vi "generate default line.vi"(8 "error in":errorcluster, 11 "operations table":T2) -> (0 "error out":errorcluster, 2 "line":T1)   [LabVIEW 2013, in "Modbus Slave editor node.lvclass"]
doc: "Platypus Framework 1.0.1.65\nNI Systems Engineering - National Instruments"
uses:
  Modbus Slave editor node.lvclass
  table reference.ctl
  table line.ctl
  <vilib>/NI/TBM Modules/modbus slave/module channel/Modbus Module Channel.lvclass
  <vilib>/NI/Tag Bus/tag/Data Type.ctl
  <vilib>/NI/TBM Modules/modbus slave/module channel/data bank type.ctl
  <vilib>/NI/Tag Bus/tag/tag descriptor.lvclass/tag descriptor.ctl
  <vilib>/NI/TBM Modules/modbus slave/module channel/Modbus Module Channel.lvclass/Modbus Module Channel.ctl
  <vilib>/NI/Tag Bus/tag/write tag name.vi
  <vilib>/NI/Tag Bus/tag/write data type.vi
  <vilib>/NI/TBM Modules/modbus slave/module channel/Write modbus type.vi
  <vilib>/NI/TBM Modules/modbus slave/module channel/Write starting address.vi
  <vilib>/NI/Tag Bus/tag/tag descriptor.lvclass
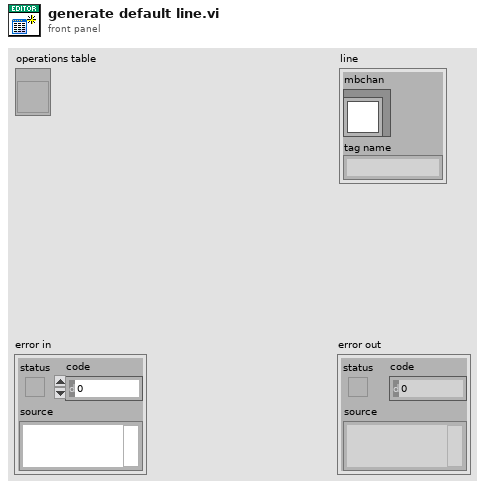
[diagram p1: front panel]
types:
  T1 = typedef "Modbus Slave editor node.lvclass/table line.ctl" = cluster{"mbchan":refnum<class "Modbus Module Channel.lvclass">, "tag name":string}
  T2 = typedef "Modbus Slave editor node.lvclass/table reference.ctl" = refnum<vi>
  T3 = typedef "Modbus Module Channel.lvclass/data bank type.ctl" = enum16{"coils", "discrete inputs", "input registers", "holding registers"}
  T4 = typedef "tag bus.lvlib/tag descriptor.lvclass/Data Type.ctl" = enum16{"Double", "Single", "I64", "I32", "I16", "I8", "U64", "U32", "U16", "U8", "Boolean", "String", "Array of Double", "Array of Single", "Array of I64", "Array of I32", "Array of I16", "Array of I8", "Array of U64", "Array of U32", "Array of U16", "Array of U8", "Array of Boolean", "Array of String"}
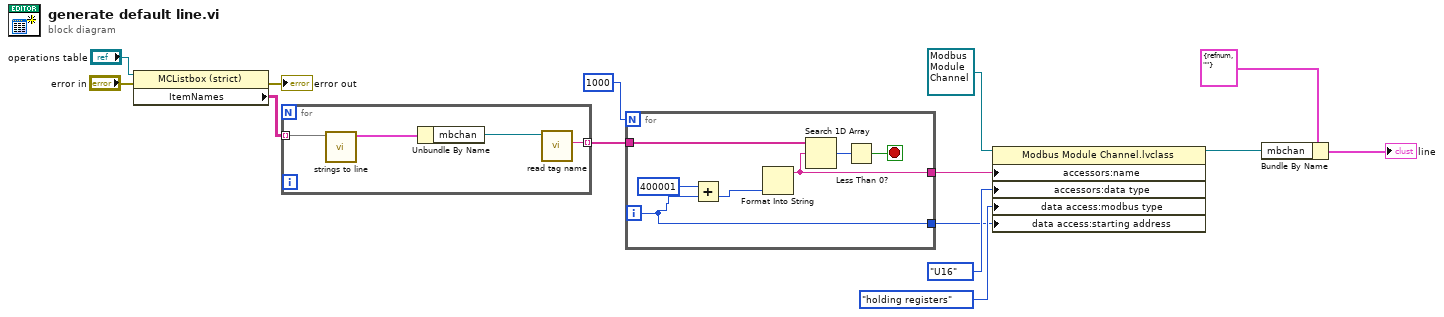
[diagram p0: block diagram]
diagram:
  n1 = property class="MCListbox (strict)"(reference="operations table", error in="error in") -> (error out=→"error out":errorcluster, "ItemNames"=w11:string[][])  [unwired: 1 out]
  n2 = for {
    tunnel: w11 -> [w18] mode=indexing
    tunnel: [w15] -> w9 mode=indexing
    n3 = call "strings to line.vi"("strings"=w18) -> ("line"=w17:T1)  [unwired: 10 in]
    n4 = Unbundle By Name(w17) -> ("mbchan"=w16:refnum<class "Modbus Module Channel.lvclass">)
    n5 = call <vilib>:"read tag name.vi"("system tag in"=w16) -> ("name"=w15:string)  [unwired: 8 in, 2 out]
  }
  n6 = for {
    N: 1000 -> [_]
    tunnel: w9 -> [w25]
    tunnel: [w22] -> w4
    tunnel: [w19] -> w1
    i -> [w19]
    stop <- w23 stop-if-true
    n7 = Add(x=400001, y=w19) -> (x+y=w21:i32)
    n8 = Format Into String(w21) -> (resulting string=w22:string)  [unwired: 3 in, 1 out]
    n9 = Search 1D Array(1D array=w25, element=w22) -> (index of element=w24:i32)  [unwired: 1 in]
    n10 = Less Than 0?(x=w24) -> (x < 0?=w23:bool)
  }
  n11 = property class="Modbus Module Channel.lvclass"(reference=refnum<class "Modbus Module Channel.lvclass"> refnum ("Modbus Module Channel"), "accessors:name"=w4, "accessors:data type"=Data_Type."U16" ("data type"), "data access:modbus type"=data_bank_type."holding registers" ("modbus type"), "data access:starting address"=w1) -> (reference out=w5:refnum<class "Modbus Module Channel.lvclass">)  [unwired: 1 in, 1 out]
  n12 = Bundle By Name(cluster=T1 {"mbchan"=refnum, "tag name"=""} ("line"), "mbchan"=w5) -> (→"line":T1)
